vi "Obtain Request Event.vi"(8 "error in (no error)":errorcluster, 10 "Create New":bool) -> (0 "error out":errorcluster, 3 "output cluster":T1)   [LabVIEW 2023, in "Head Worker.lvclass"]
uses:
  Head Worker.lvclass
  Type Def/Event Data.ctl
  <vilib>/gRPC/LabVIEW gRPC Servicer/ServiceBase/ServiceBase.lvclass
  Generated_server/RPC Service/streamai/streamai.lvclass
panel:
  # "Connector Pane"
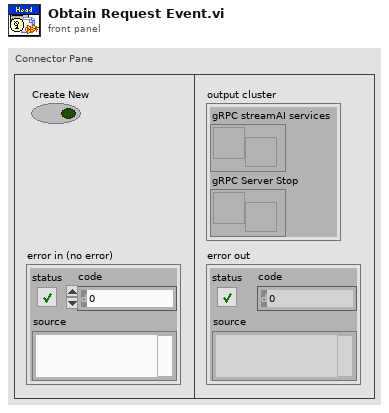
[diagram p1: front panel]
types:
  T1 = typedef "Head Worker.lvclass/Event Data.ctl" = cluster{"gRPC streamAI services":refnum<user-event>, "gRPC Server Stop":refnum<user-event>}
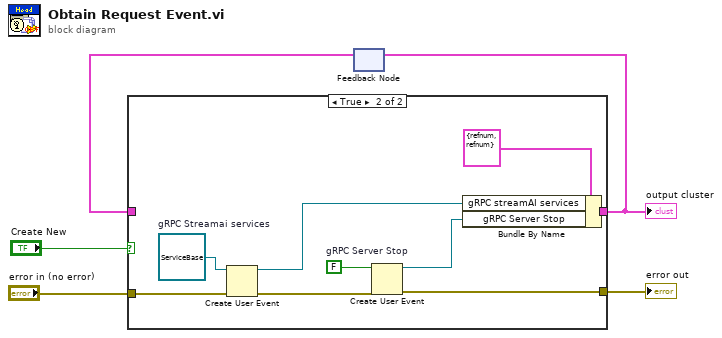
[diagram p0: block diagram]
diagram:
  n1 = feedback #1() -> (w2:T1)  [unwired: 1 in]
  n2 = case shown="True" "Create New" {
    tunnel: [w6 w10] -> w5
    tunnel: "error in (no error)" -> [w6 w9]
    tunnel: [w7 w8] -> w3
    tunnel: w2 -> [w7 _]
    frame False {
    }
    frame True {
      w15 = FALSE  # gRPC Server Stop
      w14 = refnum<class "ServiceBase.lvclass"> refnum  # gRPC Streamai services
      n3 = Create User Event(user event datatype=w14, error in=w9) -> (user event=w12:refnum<user-event>, error out=w16:errorcluster)
      n4 = Create User Event(user event datatype=w15, error in=w16) -> (user event=w13:refnum<user-event>, error out=w10:errorcluster)
      n5 = Bundle By Name(cluster=T1 {"gRPC streamAI services"=refnum, "gRPC Server Stop"=refnum} ("output cluster"), "gRPC streamAI services"=w12, "gRPC Server Stop"=w13) -> (w8:T1)
    }
  }
  "output cluster" <- w3
  "error out" <- w5
  n6 = feedback-in #1(w3) -> ()
